vi "MakeArrayTD (hid_t).vi"(7 "Use Cache":bool, 8 "error in (no error)":errorcluster, 9 "Type":enum16{"File", "Memory"}(ring)=enum."Memory", 10 "rank":i16, 11 "Element type_id":T1) -> (0 "error out":errorcluster, 2 "Default Data":string, 3 "td":i16[](array[numeric]), 4 "Description":string)   [LabVIEW 2017]
uses:
  <vilib>/UPVI/lvhdf5/library.llb/HDF5 Ref.ctl
  <userlib>/_OpenG.lib/lvdata/lvdata.llb/Type Descriptor Enumeration__ogtk.ctl
panel:
  # "LVHDF5 Toolkit\nCopyright (c) 2005-2013 by Jason D. Sommerville\nCopyright (c) 2014 by UPVI, LLC.\n\nThis use and distribution of this file is governed by the terms found in \nLICENSE.txt distributed with this toolkit and installed at\n <user.lib>\\_lvhdf5\\LICENSE.txt"
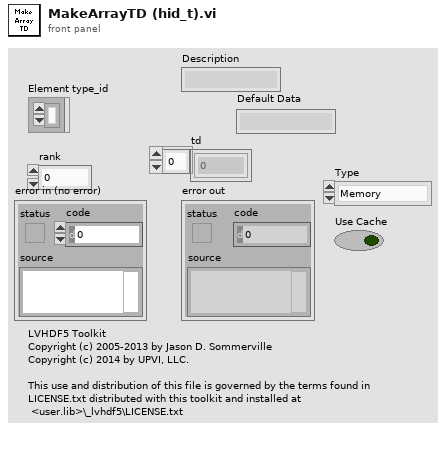
[diagram p1: front panel]
types:
  T1 = typedef "HDF5 Ref.ctl" = refnum<k1>
  T2 = typedef "Type Descriptor Enumeration__ogtk.ctl" = enum8{"<Null>", "I8", "I16", "I32", "I64", "U8", "U16", "U32", "U64", "SGL", "DBL", "EXT", "CSG", "CDB", "CXT", "0x0F", "0x10", "0x11", "0x12", "0x13", "0x14", "Enum U8", "Enum U16", "Enum U32", "Enum U64", "SGL PQ", "DBL PQ", "EXT PQ", "CSG PQ", "CDB PQ", "CXT PQ", "0x1F", "0x20", "Boolean", "0x22", "0x23", "0x24", "0x25", "0x26", "0x27", "0x28", "0x29", "0x2A", "0x2B", "0x2C", "0x2D", "0x2E", "0x2F", "String", "0x31", "Path", "Pict", "0x34", "0x35", "0x36", "DAQ", "0x38", "0x39", "0x3A", "0x3B", "0x3C", "0x3D", "0x3E", "0x3F", "Array", "0x41", "0x42", "0x43", "0x44", "0x45", "0x46", "0x47", "0x48", "0x49", "0x4A", "0x4B", "0x4C", "0x4D", "0x4E", "0x4F", "Cluster", "0x51", "0x52", "Variant", "Waveform", "0x55", "0x56", "0x57", "0x58", "0x59", "0x5A", "0x5B", "0x5C", "0x5D", "0x5E", "0x5F", "0x60", "0x61", "0x62", "0x63", "0x64", "0x65", "0x66", "0x67", "0x68", "0x69", "0x6A", "0x6B", "0x6C", "0x6D", "0x6E", "0x6F", "Refnum"}
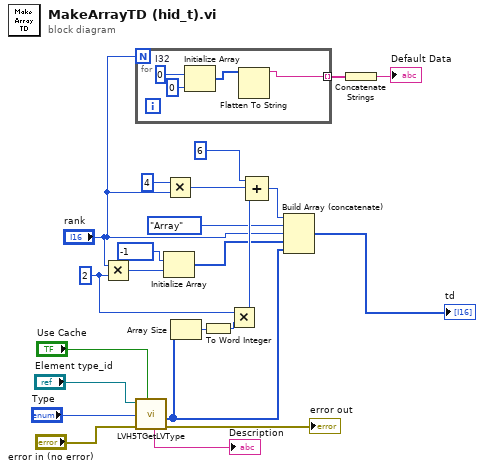
[diagram p0: block diagram]
diagram:
  w16 = i16 2 ("y")
  n1 = Multiply(x="rank", y=w16) -> (x*y=w12:i16)
  n2 = for {
    N: "rank" -> [_]
    tunnel: [w24] -> w4 mode=indexing
    w27 = 0  # I32
    n3 = Initialize Array(w27, 0 ("dimension size")) -> (w25:i32[])
    n4 = Flatten To String(anything=w25) -> (data string=w24:string)  [unwired: 3 in, 2 out]
  }
  n5 = call <vilib>:"LVH5TGetLVType.vi"("Don't use cache"="Use Cache", "error in (no error)"="error in (no error)", "Type"="Type", "HDF5 Type Ref"="Element type_id") -> ("error out"=→"error out":errorcluster, "Type String"=w21:i16[], "Description"=→"Description":string)  [unwired: 3 in, 2 out]
  n6 = Initialize Array(i16 -1 ("y"), w12) -> (w14:i16[])
  n7 = Multiply(x=i16 4, y="rank") -> (x*y=w18:i16)
  n8 = Array Size(array=w21) -> (size(s)=w15:i32)
  n9 = To Word Integer(number=w15) -> (16bit integer=w20:i16)
  n10 = Multiply(x=w16, y=w20) -> (x*y=w19:i16)
  n11 = Compound Arithmetic op=ADD(i16 6, w18, w19) -> (w22:i16)
  n12 = Build Array (concatenate)(w22, Type_Descriptor_Enumeration__ogtk."Array" ("Type Descriptor Enumeration"), "rank", w14, w21) -> (→"td":i16[])
  n13 = Concatenate Strings(w4) -> (→"Default Data":string)
